vi "Generate Macro Tree.vi"() -> ()   [LabVIEW 2012]
doc: "SciScan 1.2 160622"
uses:
  Custom Controls and Typedefs/Macro_CommandStruct.ctl
  Custom Controls and Typedefs/Macro_Action_List.ctl
  Custom Controls and Typedefs/Macro_ArgumentStruct.ctl
panel:
  out "Edit Tree Items:Add Item":string
  in  "Tree":string(tree)
  in  "Macro Array IN":T1[](array[typedef])
  in  "Tree Refnum":refnum<vi>
  out "Error Out":errorcluster
  in  "Error In":errorcluster
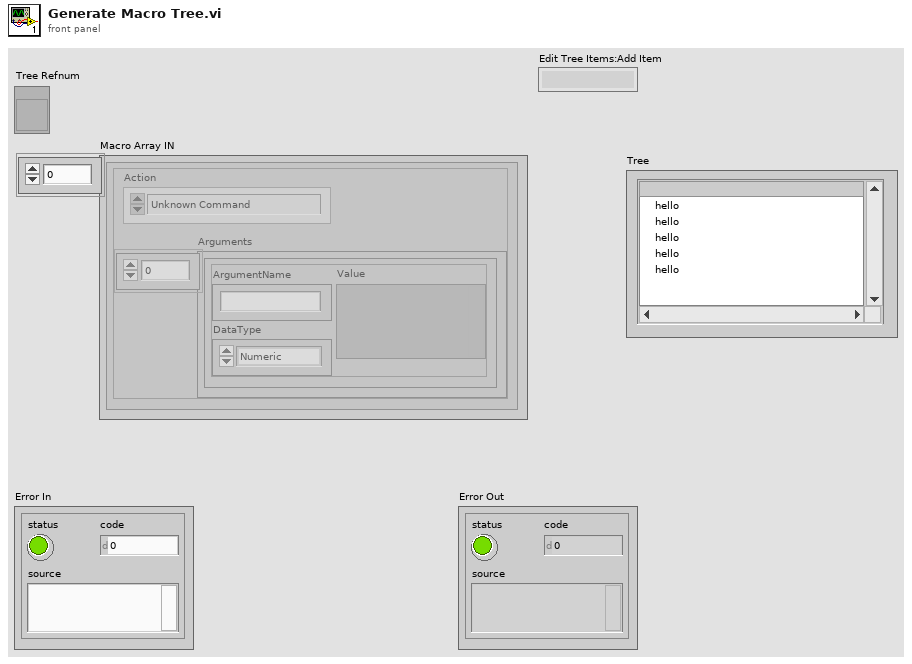
[diagram p1: front panel]
types:
  T1 = typedef "Macro_CommandStruct.ctl" = cluster{"Action":T2, "Arguments":T3[]}
  T2 = typedef "Macro_Action_List.ctl" = enum16{"Unknown Command", "2D.Frame.Scan", "2D.Line.Scan", "Load.Settings.File", "Move.To.Position", "Pause", "Z.Stack", "LOOP.Start", "LOOP.End", "Record", "Fast.Z", "Generic", "Slow.Z", "Tiling", "Preset.End"}
  T3 = typedef "Macro_ArgumentStruct.ctl" = cluster{"ArgumentName":string, "DataType":enum16{"Numeric", "String"}, "Value":variant}
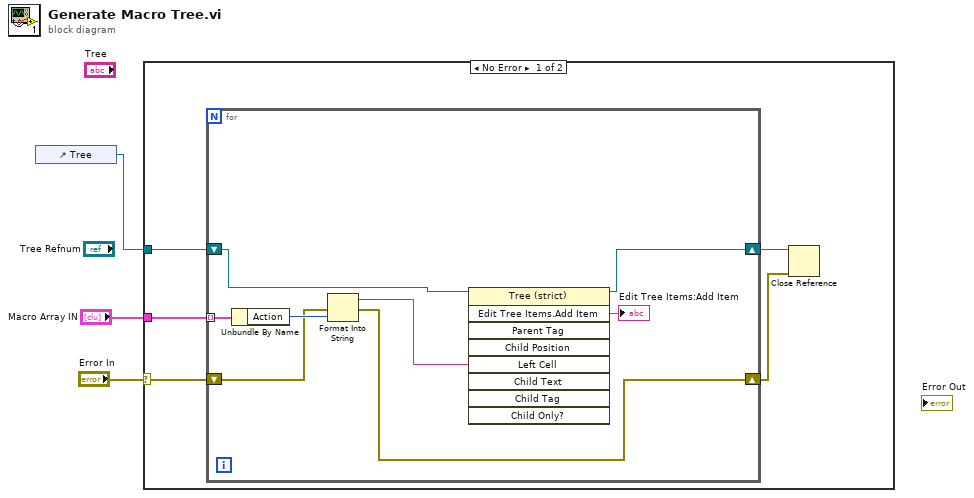
[diagram p0: block diagram]
diagram:
  n1 = control-ref of="Tree"() -> (w1:refnum<vi>)
  n2 = case shown="No Error" "Error In" {
    selector: "Error In" -> [w7 _]
    tunnel: "Macro Array IN" -> [w8 _]
    tunnel: w1 -> [w6 _]
    frame No Error {
      n3 = for {
        tunnel: w8 -> [w16] mode=indexing
        shift-right: [w13] -> w4
        shift-left: w7 -> [w14]
        shift-right: [w12] -> w5
        shift-left: w6 -> [w10]
        n4 = Unbundle By Name(w16) -> ("Action"=w15:T2)
        n5 = Format Into String(error in=w14, w15) -> (resulting string=w9:string, error out=w13:errorcluster)  [unwired: 2 in]
        n6 = invoke class="Tree (strict)" method="Edit Tree Items.Add Item"(reference=w10, "Left Cell"=w9) -> (reference out=w12:refnum<vi>, "Edit Tree Items:Add Item"=→"Edit Tree Items:Add Item":string)  [unwired: 7 in, 7 out]
      }
      n7 = Close Reference(reference=w5, error in (no error)=w4) -> ()  [unwired: 1 out]
    }
    frame Error {
    }
  }
